vi "Read salTopicEventRefnum.vi"(11 "SALCommunicator in":refnum<class "SALCommunicatorDL.lvclass">) -> (2 "salTopicEventRefnum":refnum<event-registration>, 3 "SALCommunicator out":refnum<class "SALCommunicatorDL.lvclass">)   [LabVIEW 2016, in "SALCommunicatorDL.lvclass"]
uses:
  SALCommunicatorDL.lvclass
  SALCommunicatorDL.lvclass/SALCommunicatorDL.ctl
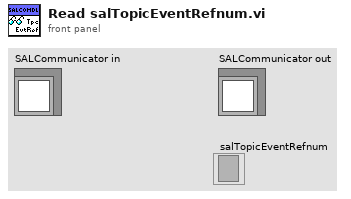
[diagram p1: front panel]
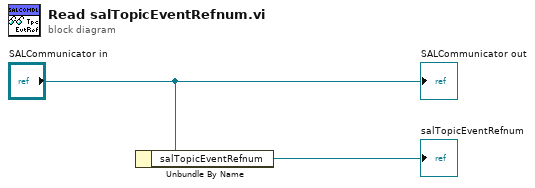
[diagram p0: block diagram]
diagram:
  n1 = Unbundle By Name("SALCommunicator in") -> ("salTopicEventRefnum"=→"salTopicEventRefnum":refnum<event-registration>)
  "SALCommunicator out" <- "SALCommunicator in"
